vi "Air MFR loff.vi"(9 "O2 Measured":dbl, 10 "O2t %":dbl, 11 "Flow rate":dbl) -> (3 "Air MFR":dbl)   [LabVIEW 2014]
uses:
  <vilib>/ptbypt/NI_PtbyPt.lvlib
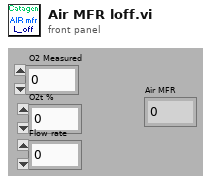
[diagram p1: front panel]
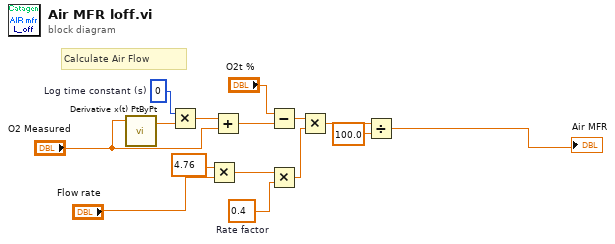
[diagram p0: block diagram]
diagram:
  w8 = 0.4  # Rate factor
  w15 = 0  # Log time constant (s)
  # "Calculate Air Flow"
  n1 = call <vilib>:"Derivative x(t) PtByPt.vi"("x"="O2 Measured") -> ("dx/dt"=w14:dbl)  [unwired: 3 in, 1 out]
  n2 = Multiply(x=w15, y=w14) -> (x*y=w13:dbl)
  n3 = Multiply(x=4.76, y="Flow rate") -> (x*y=w9:dbl)
  n4 = Add(x=w13, y="O2 Measured") -> (x+y=w12:dbl)
  n5 = Subtract(x="O2t %", y=w12) -> (x-y=w11:dbl)
  n6 = Multiply(x=w9, y=w8) -> (x*y=w7:dbl)
  n7 = Multiply(x=w11, y=w7) -> (x*y=w6:dbl)
  n8 = Divide(x=w6, y=100.0) -> (x/y=→"Air MFR":dbl)
